vi "Start VI.vi"(1 "错误输入（无错误）":errorcluster, 2 "VI名称或相对路径":string) -> (0 "error out":errorcluster)   [LabVIEW 2013]
panel:
  # "启动调用该VI的，文件夹下的一个VI"
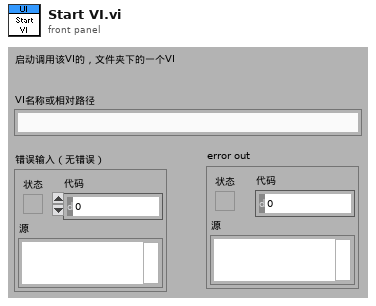
[diagram p1: front panel]
types:
  T1 = enum32{"Bad", "Idle", "Run top level", "Running"}
  T2 = enum32{"Invalid", "Standard", "Closed", "Hidden", "Minimized", "Maximized"}
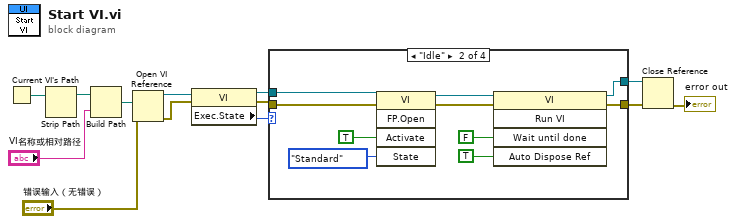
[diagram p0: block diagram]
diagram:
  n1 = Current VI's Path() -> (path=w2:path)
  n2 = Strip Path(path=w2) -> (stripped path=w3:path)  [unwired: 1 out]
  n3 = Build Path(base path=w3, name or relative path="VI名称或相对路径") -> (appended path=w4:path)
  n4 = Open VI Reference(vi path=w4, error in (no error)="错误输入（无错误）") -> (vi reference=w10:refnum<vi>, error out=w12:errorcluster)  [unwired: 4 in]
  n5 = property class="VI"(reference=w10, error in=w12) -> (reference out=w11:refnum<vi>, error out=w13:errorcluster, "Exec.State"=w9:T1)
  n6 = case shown="\"Idle\"" w9 {
    tunnel: w11 -> [w15 w23 w27 w29]
    tunnel: [w15 w18 w27 w29] -> w6
    tunnel: [w14 w17 w26 w28] -> w8
    tunnel: w13 -> [w14 w16 w26 w28]
    frame "Bad", Default {
    }
    frame "Idle" {
      n7 = invoke class="VI" method="FP.Open"(reference=w23, error in=w16, "Activate"=TRUE ("激活？"), "State"=T2."Standard" ("状态")) -> (reference out=w22:refnum<vi>, error out=w21:errorcluster)  [unwired: 1 in, 3 out]
      n8 = invoke class="VI" method="Run VI"(reference=w22, error in=w21, "Wait until done"=FALSE ("结束前等待"), "Auto Dispose Ref"=TRUE ("自动销毁引用")) -> (reference out=w18:refnum<vi>, error out=w17:errorcluster)  [unwired: 1 in, 3 out]
    }
    frame "Run top level" {
    }
    frame "Running" {
    }
  }
  n9 = Close Reference(reference=w6, error in (no error)=w8) -> (error out=→"error out":errorcluster)
